vi "get_intensity_modifier.vi"(8 "error in (no error)":errorcluster, 11 "ScanHeadAK130114ResonanceFlexRIO in":refnum<class "ScanHeadAK130114ResonanceFlexRIO.lvclass">) -> (0 "error out":errorcluster, 2 "intensity modifier":refnum<class "GenericAnalogOut.lvclass">, 3 "ScanHeadAK130114ResonanceFlexRIO out":refnum<class "ScanHeadAK130114ResonanceFlexRIO.lvclass">)   [LabVIEW 2010, in "ScanHeadAK130114ResonanceFlexRIO.lvclass"]
uses:
  ScanHeadAK130114ResonanceFlexRIO.lvclass
  AnalogOut/GenericAnalogOut/GenericAnalogOut/GenericAnalogOut.lvclass
  ScanHeadAK130114ResonanceFlexRIO.lvclass/ScanHeadAK130114ResonanceFlexRIO.ctl
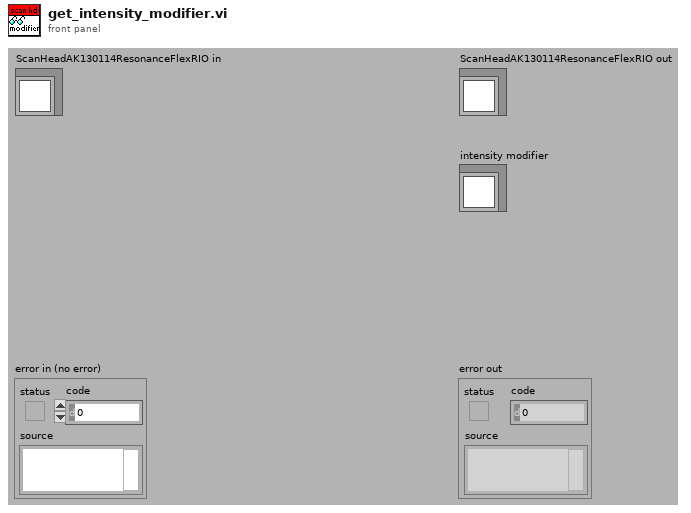
[diagram p1: front panel]
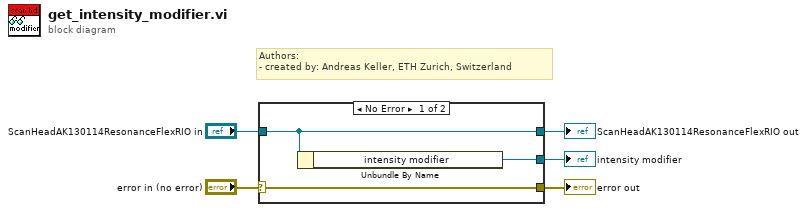
[diagram p0: block diagram]
diagram:
  # "Authors: \n- created by: Andreas Keller, ETH Zurich, Switzerland"
  n1 = case shown="No Error" "error in (no error)" {
    selector: "error in (no error)" -> [w8 w10]
    tunnel: [w8 w10] -> w4
    tunnel: [w7 w9] -> w2
    tunnel: "ScanHeadAK130114ResonanceFlexRIO in" -> [w7 w9]
    tunnel: [w6 _] -> w1
    frame No Error {
      n2 = Unbundle By Name(w7) -> ("intensity modifier"=w6:refnum<class "GenericAnalogOut.lvclass">)
    }
    frame Error {
    }
  }
  "error out" <- w4
  "ScanHeadAK130114ResonanceFlexRIO out" <- w2
  "intensity modifier" <- w1
